vi "setRightClickMenu.vi"(7 "Config Cluster":T1, 8 "error in":errorcluster, 10 "Coords":T2, 11 "MenuRef":refnum<k9>) -> (0 "error out":errorcluster)   [LabVIEW 2010]
uses:
  <vilib>/Utility/miscctls.llb/LVPoint32TypeDef.ctl
  Config cluster.ctl
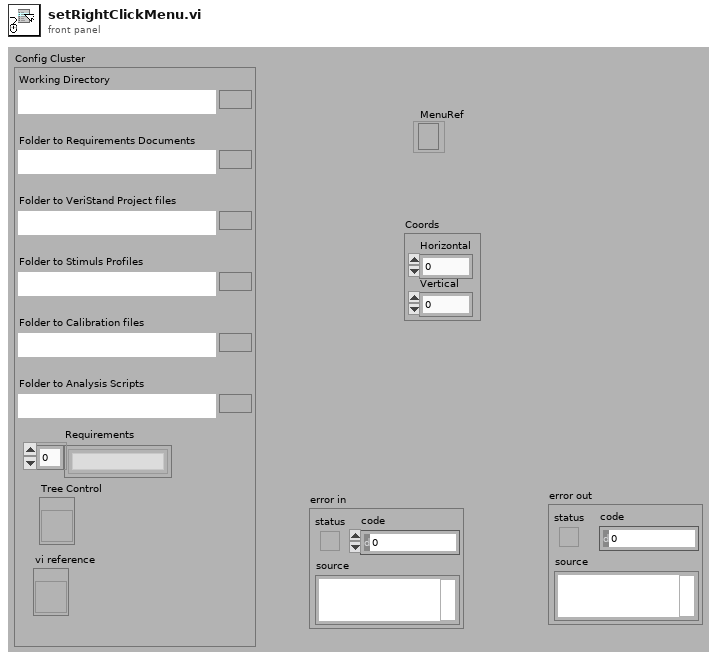
[diagram p1: front panel]
types:
  T1 = typedef "Config cluster.ctl" = cluster{"Working Directory":path, "Folder to Requirements Documents":path, "Folder to VeriStand Project files":path, "Folder to Stimuls Profiles":path, "Folder to Calibration files":path, "Folder to Analysis Scripts":path, "Requirements":string[], "Tree Control":refnum<vi>, "vi reference":refnum<vi>}
  T2 = typedef "LVPoint32TypeDef.ctl" = cluster{"Horizontal":i32, "Vertical":i32}
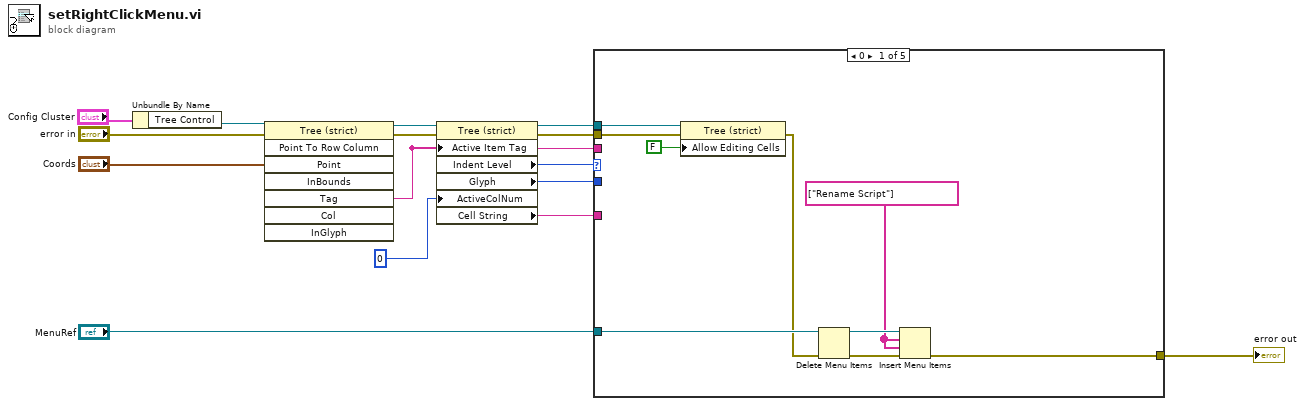
[diagram p0: block diagram]
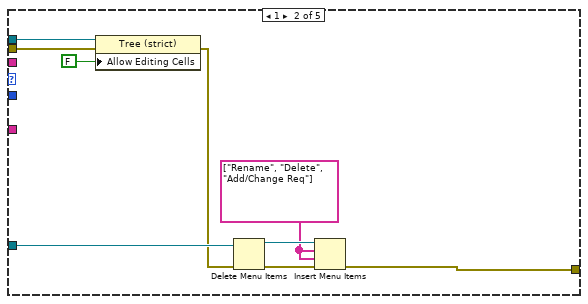
[diagram p2: hidden frame]
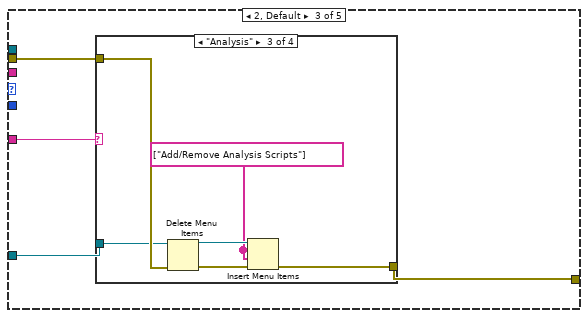
[diagram p3: hidden frame]
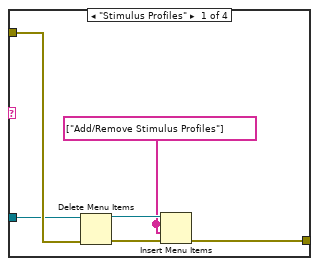
[diagram p4: hidden frame]
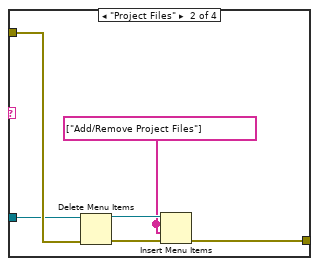
[diagram p5: hidden frame]
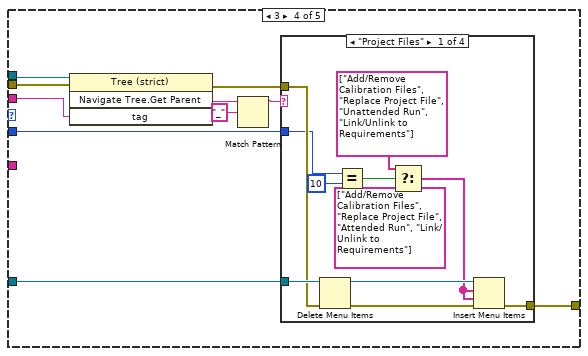
[diagram p7: hidden frame]
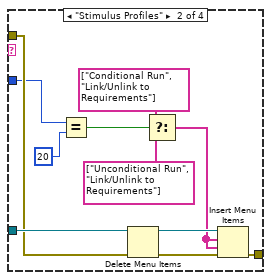
[diagram p8: hidden frame]
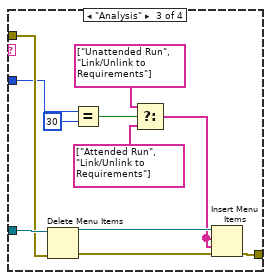
[diagram p9: hidden frame]
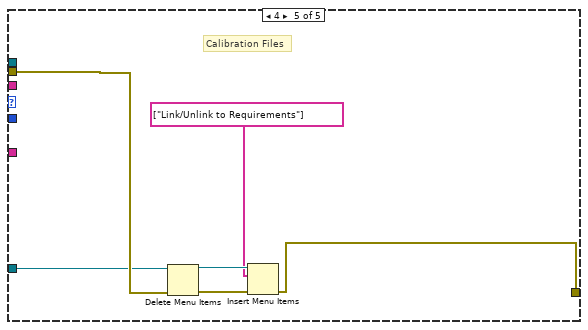
[diagram p11: hidden frame]
diagram:
  n1 = Unbundle By Name("Config Cluster") -> ("Tree Control"=w1:refnum<vi>)
  n2 = invoke class="Tree (strict)" method="Point To Row Column"(reference=w1, error in="error in", "Point"="Coords") -> (reference out=w4:refnum<vi>, error out=w8:errorcluster, "Tag"=w12:string)  [unwired: 5 in, 5 out]
  n3 = property class="Tree (strict)"(reference=w4, error in=w8, "Active Item Tag"=w12, "ActiveColNum"=0 ("Active Cell:Active Column Number")) -> (reference out=w6:refnum<vi>, error out=w9:errorcluster, "Indent Level"=w5:i32, "Glyph"=w13:i32, "Cell String"=w14:string)
  n4 = case shown="0" w5 {
    tunnel: "MenuRef" -> [w24 w33 w36 w63 w105]
    tunnel: w6 -> [w21 w30 _ w65 _]
    tunnel: w9 -> [w19 w28 w37 w66 w106]
    tunnel: [w17 w26 w35 w61 w104] -> w10
    tunnel: w12 -> [_ _ _ w64 _]
    tunnel: w13 -> [_ _ _ w57 _]
    tunnel: w14 -> [_ _ w34 _ _]
    frame 0 {
      w16 = string[] ["Rename Script"] ("item names")
      n5 = property class="Tree (strict)"(reference=w21, error in=w19, "Allow Editing Cells"=FALSE) -> (error out=w18:errorcluster)  [unwired: 1 out]
      n6 = Delete Menu Items(6:w18, 9:w24) -> (0:w22:errorcluster, 3:w23:refnum<k9>)  [unwired: 2 in]
      n7 = Insert Menu Items(6:w22, 7:w16, 8:w16, 9:w23) -> (0:w17:errorcluster)  [unwired: 2 in, 2 out]
    }
    frame 1 {
      w25 = string[] ["Rename", "Delete", "Add/Change Req"] ("item names")
      n8 = property class="Tree (strict)"(reference=w30, error in=w28, "Allow Editing Cells"=FALSE) -> (error out=w27:errorcluster)  [unwired: 1 out]
      n9 = Delete Menu Items(6:w27, 9:w33) -> (0:w31:errorcluster, 3:w32:refnum<k9>)  [unwired: 2 in]
      n10 = Insert Menu Items(6:w31, 7:w25, 8:w25, 9:w32) -> (0:w26:errorcluster)  [unwired: 2 in, 2 out]
    }
    frame 2, Default {
      n11 = case shown="\"Analysis\"" w34 {
        tunnel: w37 -> [w43 w49 w55 w56]
        tunnel: [w40 w46 w52 w56] -> w35
        tunnel: w36 -> [w39 w45 w51 _]
        frame "Stimulus Profiles" {
          w38 = string[] ["Add/Remove Stimulus Profiles"] ("item names")
          n12 = Delete Menu Items(6:w43, 9:w39) -> (0:w42:errorcluster, 3:w41:refnum<k9>)  [unwired: 2 in]
          n13 = Insert Menu Items(6:w42, 7:w38, 8:w38, 9:w41) -> (0:w40:errorcluster)  [unwired: 2 in, 2 out]
        }
        frame "Project Files" {
          w44 = string[] ["Add/Remove Project Files"] ("item names")
          n14 = Delete Menu Items(6:w49, 9:w45) -> (0:w48:errorcluster, 3:w47:refnum<k9>)  [unwired: 2 in]
          n15 = Insert Menu Items(6:w48, 7:w44, 8:w44, 9:w47) -> (0:w46:errorcluster)  [unwired: 2 in, 2 out]
        }
        frame "Analysis" {
          w50 = string[] ["Add/Remove Analysis Scripts"] ("item names")
          n16 = Delete Menu Items(6:w55, 9:w51) -> (0:w54:errorcluster, 3:w53:refnum<k9>)  [unwired: 2 in]
          n17 = Insert Menu Items(6:w54, 7:w50, 8:w50, 9:w53) -> (0:w52:errorcluster)  [unwired: 2 in, 2 out]
        }
        frame Default {
        }
      }
    }
    frame 3 {
      n18 = invoke class="Tree (strict)" method="Navigate Tree.Get Parent"(reference=w65, error in=w66, "tag"=w64) -> (error out=w62:errorcluster, "Navigate Tree:Get Parent"=w60:string)  [unwired: 1 in, 2 out]
      n19 = Match Pattern(string=w60, regular expression="_") -> (before substring=w59:string)  [unwired: 1 in, 3 out]
      n20 = case shown="\"Project Files\"" w59 {
        tunnel: w63 -> [w77 w88 w99 _]
        tunnel: w62 -> [w76 w87 w98 w100]
        tunnel: [w73 w84 w95 w100] -> w61
        tunnel: w57 -> [w69 w79 w91 _]
        frame "Project Files" {
          n21 = Delete Menu Items(6:w76, 9:w77) -> (0:w75:errorcluster, 3:w74:refnum<k9>)  [unwired: 2 in]
          n22 = Equal?(x=w69, y=10) -> (x = y?=w70:bool)
          n23 = Select(t=string[] ["Add/Remove Calibration Files", "Replace Project File", "Unattended Run", "Link/Unlink to Requirements"] ("item names"), s=w70, f=string[] ["Add/Remove Calibration Files", "Replace Project File", "Attended Run", "Link/Unlink to Requirements"] ("item names")) -> (s? t:f=w67:string[])
          n24 = Insert Menu Items(6:w75, 7:w67, 8:w67, 9:w74) -> (0:w73:errorcluster)  [unwired: 2 in, 2 out]
        }
        frame "Stimulus Profiles" {
          n25 = Equal?(x=w79, y=20) -> (x = y?=w81:bool)
          n26 = Delete Menu Items(6:w87, 9:w88) -> (0:w86:errorcluster, 3:w85:refnum<k9>)  [unwired: 2 in]
          n27 = Select(t=string[] ["Conditional Run", "Link/Unlink to Requirements"] ("item names"), s=w81, f=string[] ["Unconditional Run", "Link/Unlink to Requirements"] ("item names")) -> (s? t:f=w78:string[])
          n28 = Insert Menu Items(6:w86, 7:w78, 8:w78, 9:w85) -> (0:w84:errorcluster)  [unwired: 2 in, 2 out]
        }
        frame "Analysis" {
          n29 = Delete Menu Items(6:w98, 9:w99) -> (0:w97:errorcluster, 3:w96:refnum<k9>)  [unwired: 2 in]
          n30 = Equal?(x=w91, y=30) -> (x = y?=w92:bool)
          n31 = Select(t=string[] ["Unattended Run", "Link/Unlink to Requirements"] ("item names"), s=w92, f=string[] ["Attended Run", "Link/Unlink to Requirements"] ("item names")) -> (s? t:f=w89:string[])
          n32 = Insert Menu Items(6:w97, 7:w89, 8:w89, 9:w96) -> (0:w95:errorcluster)  [unwired: 2 in, 2 out]
        }
        frame Default {
        }
      }
    }
    frame 4 {
      # "Calibration Files"
      n33 = Delete Menu Items(6:w106, 9:w105) -> (0:w103:errorcluster, 3:w102:refnum<k9>)  [unwired: 2 in]
      n34 = Insert Menu Items(6:w103, 8:string[] ["Link/Unlink to Requirements"] ("item names"), 9:w102) -> (0:w104:errorcluster)  [unwired: 3 in, 2 out]
    }
  }
  "error out" <- w10
